vi "GetClassAttribute.vi"(5 "error in (no error)":errorcluster) -> (12 "created new":bool, 15 "Int":i32, 16 "ArrayInt":i32[](array[numeric]), 19 "error out":errorcluster)   [LabVIEW 2010, in "G#BaseClass1.lvclass"]
uses:
  G#BaseClass1.lvclass
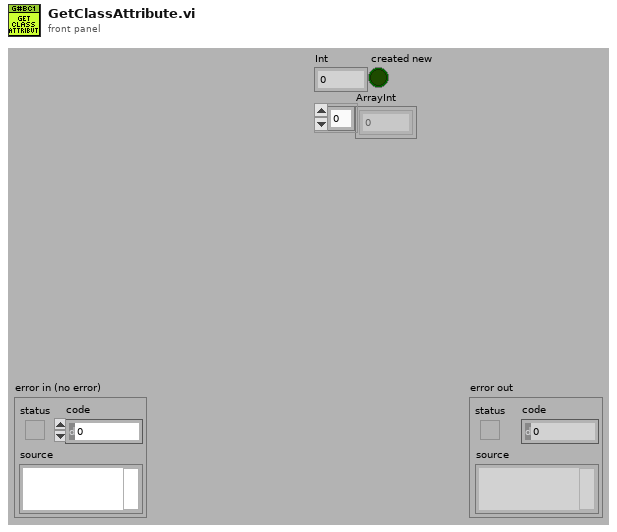
[diagram p1: front panel]
types:
  T1 = typedef "G#BaseClass1.lvclass/ClassAttributes.ctl" = cluster{"Int":i32, "ArrayInt":i32[]}
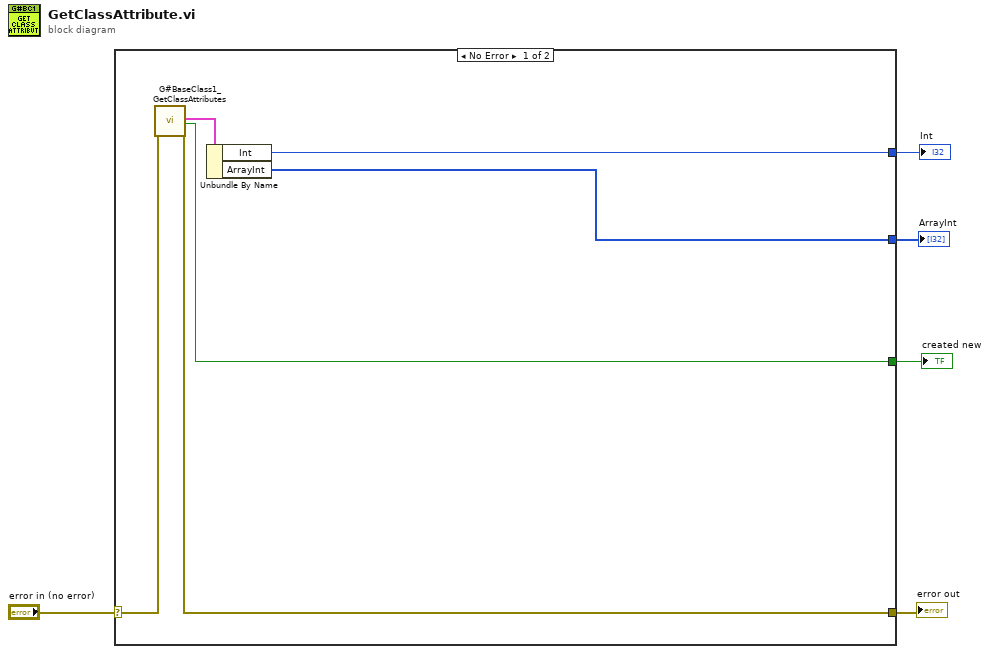
[diagram p0: block diagram]
diagram:
  n1 = case shown="No Error" "error in (no error)" {
    selector: "error in (no error)" -> [w11 w12]
    tunnel: [w10 w12] -> w4
    tunnel: [w8 _] -> w3
    tunnel: [w7 _] -> w2
    tunnel: [w6 _] -> w1
    frame No Error {
      n2 = call "G#BaseClass1_GetClassAttributes.vi"("error in (no error)"=w11) -> ("class attributes"=w9:T1, "created new?"=w6:bool, "error out"=w10:errorcluster)  [unwired: 15 in, 1 out]
      n3 = Unbundle By Name(w9) -> ("Int"=w8:i32, "ArrayInt"=w7:i32[])
    }
    frame Error {
    }
  }
  "error out" <- w4
  "Int" <- w3
  "ArrayInt" <- w2
  "created new" <- w1
